vi "string subset 7.vi"() -> ()   [LabVIEW 2025]
panel:
  out "o/p indicator":string
  in  "INPUT string":string
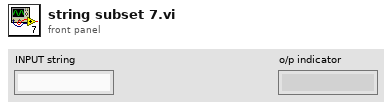
[diagram p1: front panel]
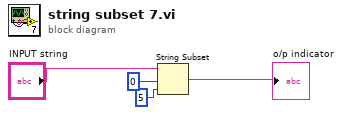
[diagram p0: block diagram]
diagram:
  n1 = String Subset(string="INPUT string", offset (0)=0, length (rest)=5) -> (substring=→"o/p indicator":string)
